vi "OLA Find Fit.vi"(8 "order":i32=3, 9 "fit fraction":dbl=0.18, 10 "ignore first":i32=5, 11 "signal":dbl[](array[numeric])) -> (1 "coefficients":dbl[](array[numeric]), 2 "fit":dbl[](array[numeric]), 3 "subtracted":dbl[](array[numeric]))   [LabVIEW 2019]
uses:
  <vilib>/Analysis/NI_AALPro.lvlib
  <vilib>/Analysis/NI_AALBase.lvlib
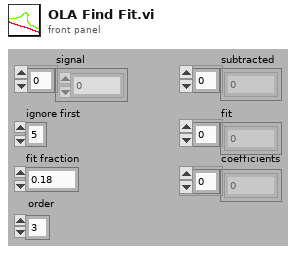
[diagram p1: front panel]
types:
  T1 = enum32{"SVD", "Givens", "Givens2", "Householder", "LU Decomposition", "Cholesky"}
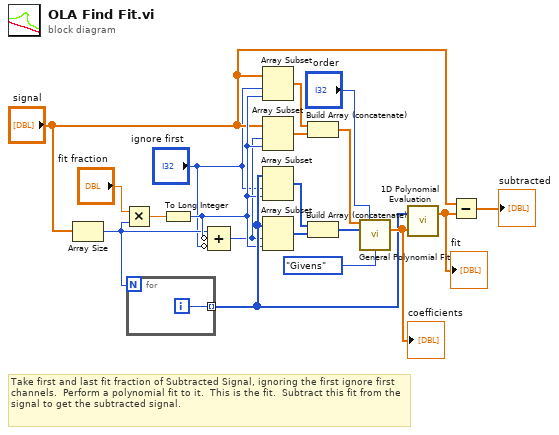
[diagram p0: block diagram]
diagram:
  # "Take first and last fit fraction of Subtracted Signal, ignoring the first ignore first channels.  Perform a polynomial fit to it.  This is the fit.  Subtract this fit from the signal to get the subtracted signal."
  n1 = Array Size(array="signal") -> (size(s)=w7:i32)
  n2 = Multiply(x="fit fraction", y=w7) -> (x*y=w19:dbl)
  n3 = for {
    N: w7 -> [_]
    tunnel: [w20] -> w13 mode=indexing
    i -> [w20]
  }
  n4 = To Long Integer(number=w19) -> (32bit integer=w9:i32)
  n5 = Compound Arithmetic op=ADD(w7, invert w9, invert "ignore first") -> (w8:i32)
  n6 = Array Subset(array="signal", index="ignore first", length=w9) -> (w18:dbl[])
  n7 = Array Subset(array="signal", index=w8, length=w9) -> (w17:dbl[])
  n8 = Array Subset(array=w13, index="ignore first", length=w9) -> (w16:i32[])
  n9 = Array Subset(array=w13, index=w8, length=w9) -> (w15:i32[])
  n10 = Build Array (concatenate)(w18, w17) -> (w12:dbl[])
  n11 = Build Array (concatenate)(w16, w15) -> (w11:i32[])
  n12 = call <vilib>:"General Polynomial Fit.vi"("Y"=w12, "polynomial order"="order", "X"=w11, "algorithm"=T1."Givens") -> ("Polynomial Coefficients"=w14:dbl[])  [unwired: 8 in, 3 out]
  "coefficients" <- w14
  n13 = call <vilib>:"1D Polynomial Evaluation.vi"("Coefficients: a"=w14, "X"=w13) -> ("Y"=w2:dbl[])  [unwired: 1 out]
  "fit" <- w2
  n14 = Subtract(x="signal", y=w2) -> (x-y=→"subtracted":dbl[])
